vi "Configure Display Format.vi"(6 "Unit (0: DBM)":i32(ring) items=["DBM", "DBMV", "DBMA", "W", "V", "A"], 8 "error in (no error)":errorcluster, 9 "Display Format (0: Magnitude Linear)":i32(ring) items=["Magnitude Linear", "Magnitude Logarithmic", "Phase", "Unwrapped phase", "Imaginary", "Real", "Polar", "Smith Chart", "Smith Admittance", "SWR", "Group Delay", "Kelvin", "Fahrenheit", "Celsius"], 10 "Channel (1)":i32=1, 11 "VISA resource name":refnum<visa-resource-name>) -> (0 "error out":errorcluster, 3 "VISA resource name out":refnum<visa-resource-name>)   [LabVIEW 2018, in "Keysight PNA Series.lvlib"]
doc: "Configures the display format for the measurement."
uses:
  Keysight PNA Series.lvlib
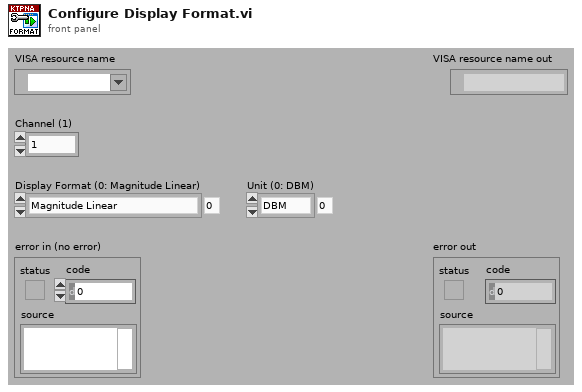
[diagram p1: front panel]
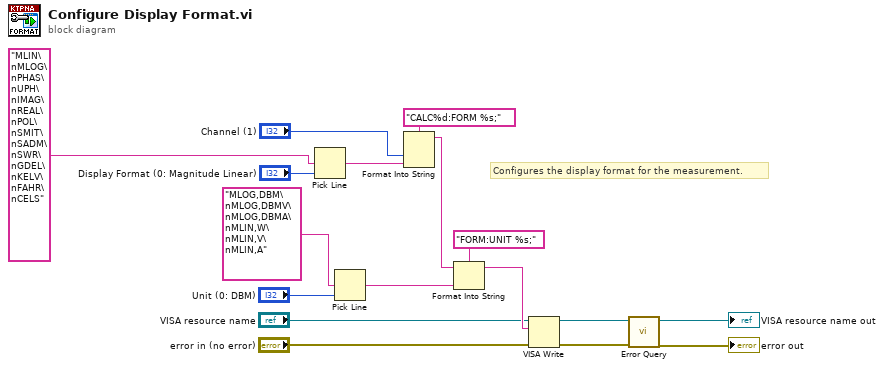
[diagram p0: block diagram]
diagram:
  # "Configures the display format for the measurement."
  n1 = Pick Line(multi-line string="MLIN\nMLOG\nPHAS\nUPH\nIMAG\nREAL\nPOL\nSMIT\nSADM\nSWR\nGDEL\nKELV\nFAHR\nCELS", line index="Display Format (0: Magnitude Linear)") -> (output string=w14:string)  [unwired: 1 in]
  n2 = Pick Line(multi-line string="MLOG,DBM\nMLOG,DBMV\nMLOG,DBMA\nMLIN,W\nMLIN,V\nMLIN,A", line index="Unit (0: DBM)") -> (output string=w2:string)  [unwired: 1 in]
  n3 = Format Into String(format string="CALC%d:FORM %s;", "Channel (1)", w14) -> (resulting string=w11:string)  [unwired: 2 in, 1 out]
  n4 = Format Into String(format string="FORM:UNIT %s;", initial string=w11, w2) -> (resulting string=w9:string)  [unwired: 1 in, 1 out]
  n5 = VISA Write(VISA resource name="VISA resource name", write buffer=w9, error in (no error)="error in (no error)") -> (VISA resource name out=w6:refnum<visa-resource-name>, error out=w5:errorcluster)  [unwired: 1 out]
  n6 = call "Error Query.vi"("error in (no error)"=w5, "VISA resource name"=w6) -> ("error out"=→"error out":errorcluster, "VISA resource name out"=→"VISA resource name out":refnum<visa-resource-name>)  [unwired: 6 in, 2 out]
